vi "Parse Text.vi"(8 "Error In":errorcluster, 11 "Parser In":refnum<class "Lexer.lvclass">) -> (0 "Error Out":errorcluster, 3 "Parser Out":refnum<class "Lexer.lvclass">)   [LabVIEW 2018, in "Toolkit.lvlib" / "Lexer.lvclass"]
uses:
  Lexer.lvclass
  Lexer.lvclass/Lexer.ctl
  Type Definitions/States.ctl
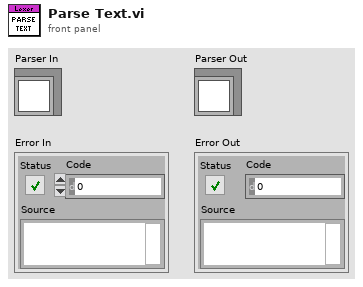
[diagram p1: front panel]
types:
  T1 = typedef "Toolkit.lvlib/Lexer.lvclass/States.ctl" = enum16{"Text", "Open Delimiter", "Tag Type", "Tag Key", "Close Delimiter"}
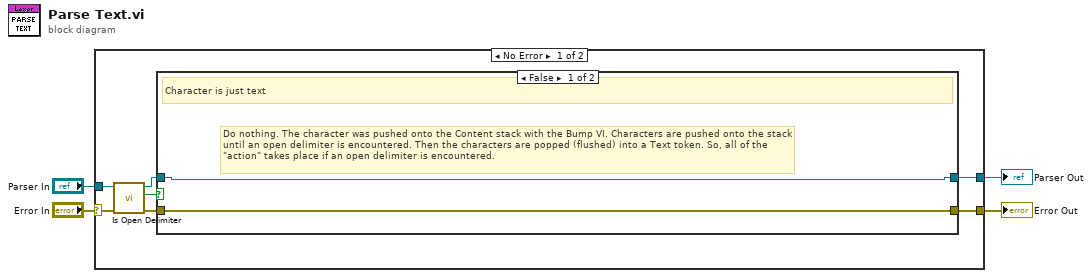
[diagram p0: block diagram]
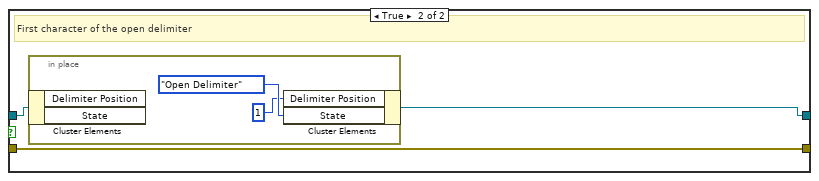
[diagram p2: hidden frame]
diagram:
  n1 = case shown="No Error" "Error In" {
    selector: "Error In" -> [w11 w20]
    tunnel: "Parser In" -> [w10 w19]
    tunnel: [w6 w19] -> w3
    tunnel: [w5 w20] -> w1
    frame No Error {
      n2 = call "Is Open Delimiter.vi"("Error In"=w11, "Parser In"=w10) -> ("Error Out"=w7:errorcluster, "Open Delimiter"=w9:bool, "Parser Out"=w8:refnum<class "Lexer.lvclass">)  [unwired: 7 in]
      n3 = case shown="False" w9 {
        tunnel: w8 -> [w12 w15]
        tunnel: w7 -> [w13 w14]
        tunnel: [w12 w16] -> w6
        tunnel: [w13 w14] -> w5
        frame False {
          # "Do nothing. The character was pushed onto the Content stack with the Bump VI. Characters are pushed onto the stack until an open delimiter is encountered. Then the characters are popped (flushed) into a Text token. So, all of the \"action\" takes place if an open delimiter is encountered."
          # "Character is just text"
        }
        frame True {
          # "First character of the open delimiter"
          n4 = in-place {
            n5 = in-place-cluster #1(w15) -> ()  [unwired: 2 out]
            n6 = in-place-cluster #1("Delimiter Position"=1, "State"=States."Open Delimiter") -> (w16:refnum<class "Lexer.lvclass">)
          }
        }
      }
    }
    frame Error {
    }
  }
  "Parser Out" <- w3
  "Error Out" <- w1
